vi "unused_getType.vi"(8 "error in (no error)":errorcluster, 11 "Decoration In":refnum<class "Decoration.lvclass">) -> (0 "error out":errorcluster, 2 "type":refnum<vi>, 3 "Decoration Out":refnum<class "Decoration.lvclass">)   [LabVIEW 2023]
uses:
  Decoration.lvclass/Decoration.ctl
  Decoration.lvclass
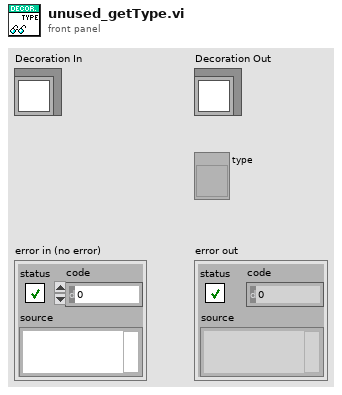
[diagram p1: front panel]
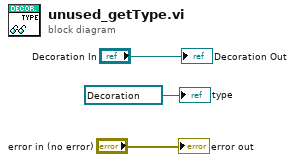
[diagram p0: block diagram]
diagram:
  "error out" <- "error in (no error)"
  "Decoration Out" <- "Decoration In"
  "type" <- refnum<vi> refnum ("type")
